vi "Set Pulse Amplitude.vi"(8 "error in (no error)":errorcluster, 9 "Amplitude":dbl=1.0, 10 "Function (0:Voltage)":u16(ring) items=["Voltage", "Current"], 11 "VISA resource name":refnum<visa-resource-name>="USB0::0x05E6::0x2461::04090176::INSTR") -> (0 "error out":errorcluster, 3 "VISA resource name out":refnum<visa-resource-name>="USB0::0x05E6::0x2461::04090176::INSTR")   [LabVIEW 2025, in "Keithley 2450.lvlib"]
doc: "This command sets the output level of the voltage or current source pulse when pulsing.\nThe sign of the source level dictates the polarity of the source. Positive values generate positive\nvoltage or current from the high terminal of the source relative to the low terminal. Negative values\ngenerate negative voltage or current from the high terminal of the source relative to the low terminal.\nIf a manual source range is selected, the level cannot exceed the specified range. For example, if the\nvoltage source is on the 2 V range, you cannot set the voltage source amplitude to 3 V. When auto\nrange is selected, the amplitude can be set to any level supported by the instrument because it will\nselect the correct range automatically when pulsing.\n\n<B>This function is only compatible with the 2461.</B>"
uses:
  Keithley 2450.lvlib
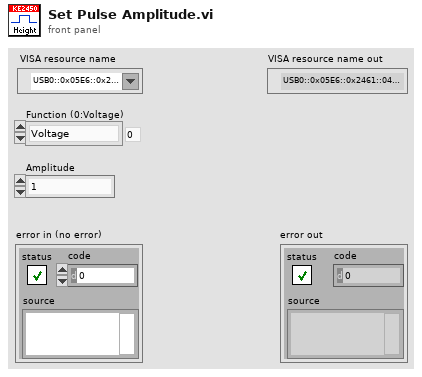
[diagram p1: front panel]
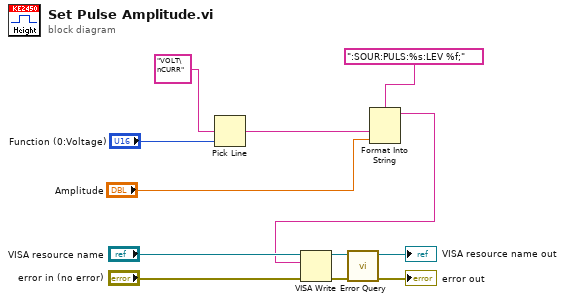
[diagram p0: block diagram]
diagram:
  n1 = Pick Line(multi-line string="VOLT\nCURR", line index="Function (0:Voltage)") -> (output string=w1:string)  [unwired: 1 in]
  n2 = Format Into String(format string=":SOUR:PULS:%s:LEV %f;" ("multi-line string"), w1, "Amplitude") -> (resulting string=w3:string)  [unwired: 2 in, 1 out]
  n3 = VISA Write(VISA resource name="VISA resource name", write buffer=w3, error in (no error)="error in (no error)") -> (VISA resource name out=w8:refnum<visa-resource-name>, error out=w7:errorcluster)  [unwired: 1 out]
  n4 = call "Error Query.vi"("error in (no error)"=w7, "VISA resource name"=w8) -> ("error out"=→"error out":errorcluster, "VISA resource name out"=→"VISA resource name out":refnum<visa-resource-name>)  [unwired: 8 out]
